vi "Create Base Queue.vi"(9 "Queue":refnum<class "Queue.lvclass">, 10 "Self Queue Alias":string) -> (0 "error out":errorcluster)   [LabVIEW 2021, in "jettl.lvlib"]
uses:
  jettl.lvlib
  Base Queue/Base Queue.lvlib
  Queue/Queue.lvclass
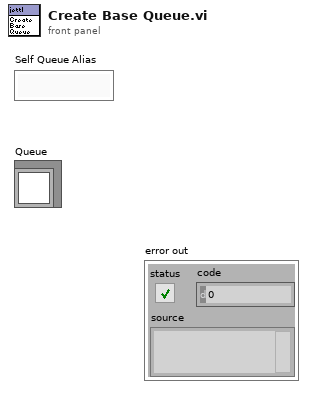
[diagram p1: front panel]
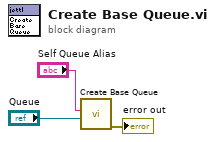
[diagram p0: block diagram]
diagram:
  n1 = call "Create Base Queue.vi"("Queue jettl"="Queue", "Alias"="Self Queue Alias") -> ("error out"=→"error out":errorcluster)  [unwired: 9 in]
